vi "FindCentroid.vi"(6 "i":u8, 8 "Plot":T1, 10 "Last PosX":dbl, 11 "New PosX":dbl) -> (0 "nearest point":i32, 1 "f Centroid":dbl, 2 "Filter line":dbl[](array[numeric]), 3 "mean":dbl, 4 "start":i32)   [LabVIEW 2022 SP3]
uses:
  <vilib>/Analysis/NI_AALBase.lvlib
  <vilib>/Analysis/baseanly.llb/Mean (DBL).vi
panel:
  out "Pts in Range":i32
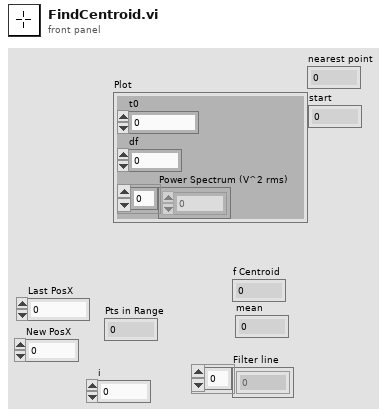
[diagram p1: front panel]
types:
  T1 = cluster{"t0":dbl, "df":dbl, "Power Spectrum (V^2 rms)":dbl[]}
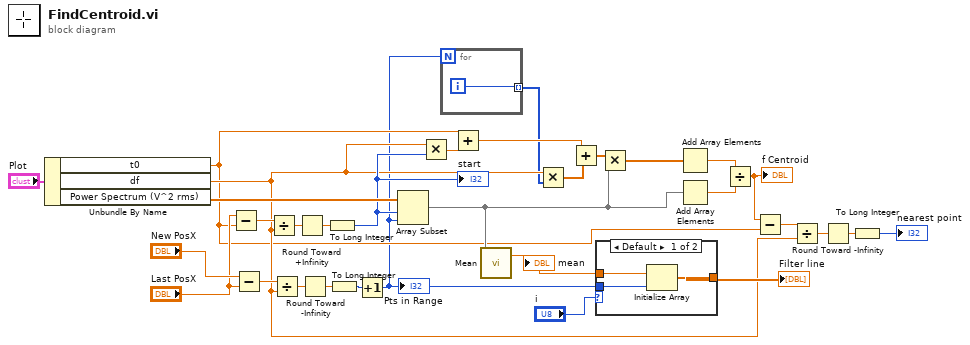
[diagram p0: block diagram]
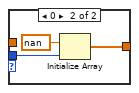
[diagram p2: hidden frame]
diagram:
  n1 = Unbundle By Name("Plot") -> ("t0"=w11:dbl, "df"=w16:dbl, "Power Spectrum (V^2 rms)"=w26:dbl[])
  n2 = Subtract(x="Last PosX", y=w11) -> (x-y=w29:dbl)
  n3 = Subtract(x="New PosX", y="Last PosX") -> (x-y=w27:dbl)
  n4 = Divide(x=w29, y=w16) -> (x/y=w32:dbl)
  n5 = Divide(x=w27, y=w16) -> (x/y=w31:dbl)
  n6 = Round Toward +Infinity(x=w32) -> (ceil(x): smallest int >= x=w24:dbl)
  n7 = Round Toward -Infinity(1:w31) -> (0:w25:dbl)
  n8 = To Long Integer(number=w24) -> (32bit integer=w22:i32)
  "start" <- w22
  n9 = To Long Integer(number=w25) -> (32bit integer=w9:i32)
  n10 = Increment(x=w9) -> (x+1=w1:i32)
  "Pts in Range" <- w1
  n11 = Array Subset(array=w26, index=w22, length=w1) -> (w19:dbl[])
  n12 = Multiply(x=w16, y=w22) -> (x*y=w21:dbl)
  n13 = for {
    N: w1 -> [_]
    tunnel: [w33] -> w3 mode=indexing
    i -> [w33]
  }
  n14 = Add(x=w11, y=w21) -> (x+y=w20:dbl)
  n15 = call-poly <vilib>:"Mean.vi"("X"=w19) -> ("mean"=w17:dbl)  [unwired: 1 out]
  "mean" <- w17
  n16 = Multiply(x=w16, y=w3) -> (x*y=w5:dbl[])
  n17 = Add(x=w20, y=w5) -> (x+y=w4:dbl[])
  n18 = case shown="Default" "i" {
    tunnel: [w36 w39] -> w18
    tunnel: w17 -> [w35 _]
    tunnel: w1 -> [w34 w38]
    frame Default {
      n19 = Initialize Array(w35, w34) -> (w36:dbl[])
    }
    frame 0 {
      n20 = Initialize Array(nan ("element"), w38) -> (w39:dbl[])
    }
  }
  "Filter line" <- w18
  n21 = Multiply(x=w4, y=w19) -> (x*y=w8:dbl[])
  n22 = Add Array Elements(numeric array=w8) -> (sum=w7:dbl)
  n23 = Add Array Elements(numeric array=w19) -> (sum=w6:dbl)
  n24 = Divide(x=w7, y=w6) -> (x/y=w12:dbl)
  "f Centroid" <- w12
  n25 = Subtract(x=w12, y=w11) -> (x-y=w10:dbl)
  n26 = Divide(x=w10, y=w16) -> (x/y=w14:dbl)
  n27 = Round Toward -Infinity(1:w14) -> (0:w15:dbl)
  n28 = To Long Integer(number=w15) -> (32bit integer=→"nearest point":i32)
